vi "Test.vi"() -> ()   [LabVIEW 2020]
uses:
  g_industrial_cam/Device Enumeration.ctl
  g_industrial_cam/Camera/Camera.lvclass/Camera.ctl
  g_industrial_cam/Buffer/Buffer.lvclass/Buffer.ctl
  g_industrial_cam/Buffer/Create from Handle.vi
  g_industrial_cam/Camera/Check Not Disconnected.vi
  <vilib>/Utility/error.llb/Error Cluster From Error Code.vi
  <vilib>/picture/picture.llb/Draw 8-Bit Pixmap.vi
  g_industrial_cam/Buffer/Buffer.lvclass
  g_industrial_cam/Camera/Camera.lvclass
panel:
  out "Waveform Chart":i32(graph)
  out "Timeout":bool
  out "Devices":T1[](array[typedef])
  in  "Picture Zoom Factor":sgl
  out "2D Picture":picture
  out "Snap Shot Count":i32
  in  "stop":bool
  out "error out":errorcluster
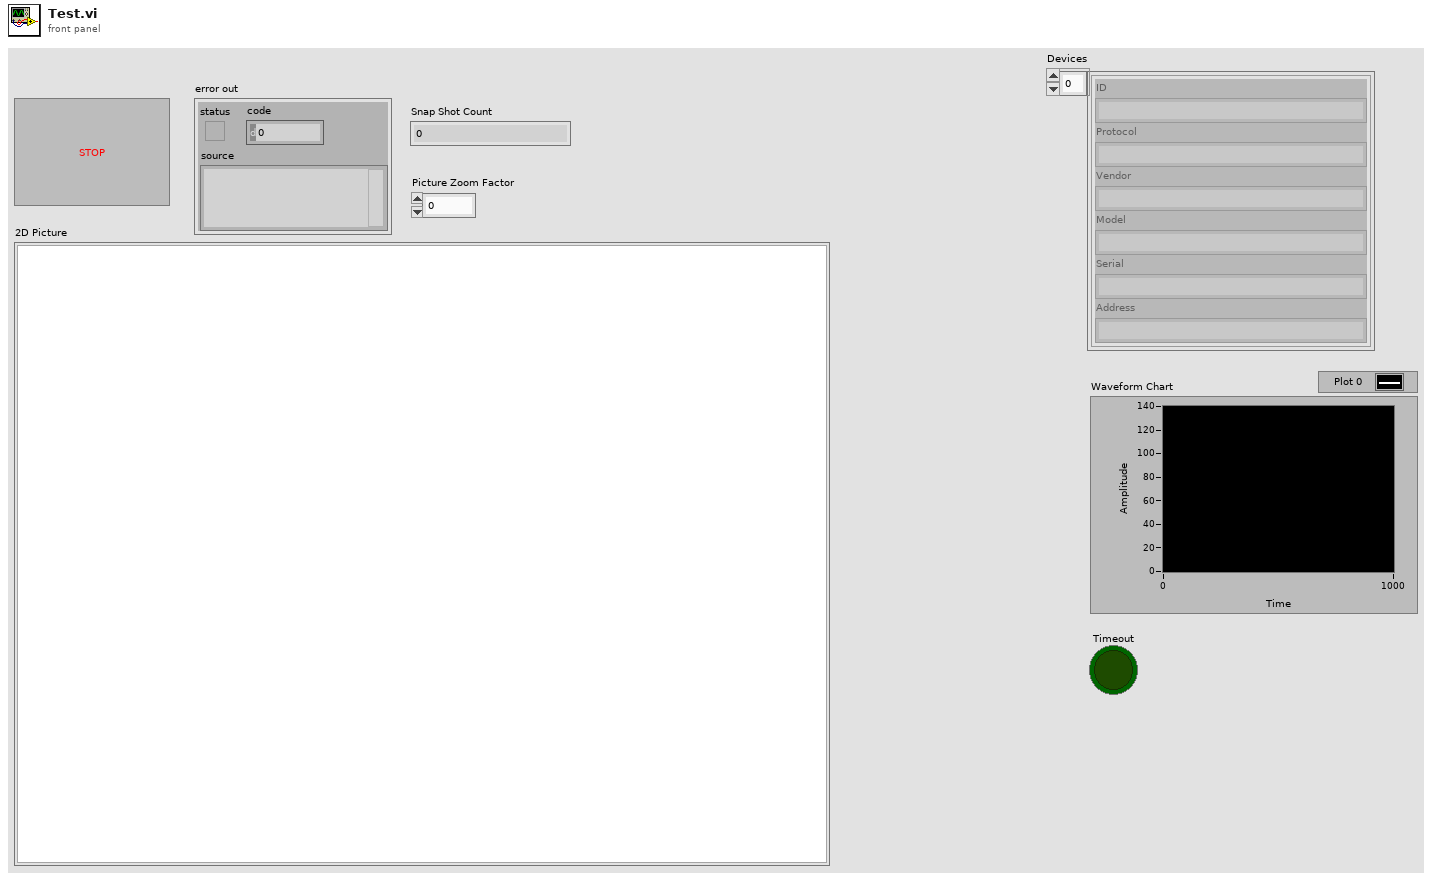
[diagram p1: front panel]
types:
  T1 = typedef "Device Enumeration.ctl" = cluster{"ID":string, "Protocol":string, "Vendor":string, "Model":string, "Serial":string, "Address":string}
  T2 = typedef "Buffer.lvclass/Image Size.ctl" = cluster{"Width":u16, "Height":u16}
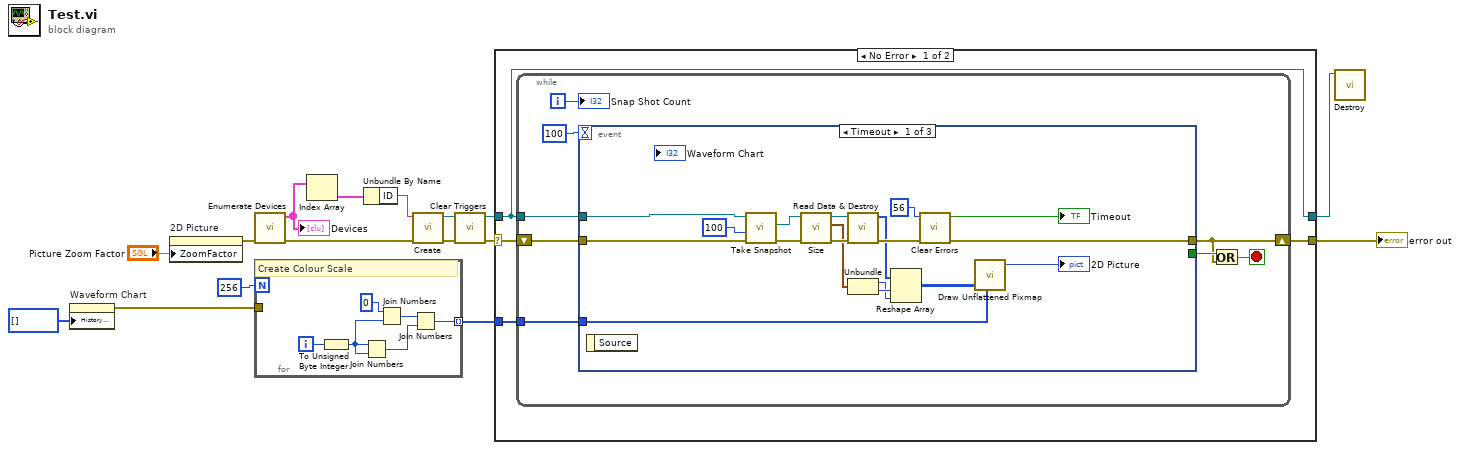
[diagram p0: block diagram]
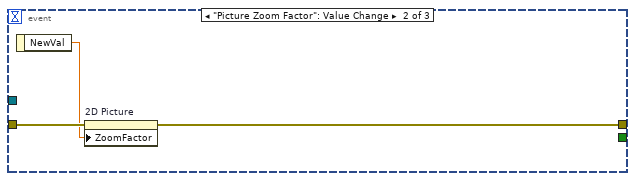
[diagram p2: hidden frame]
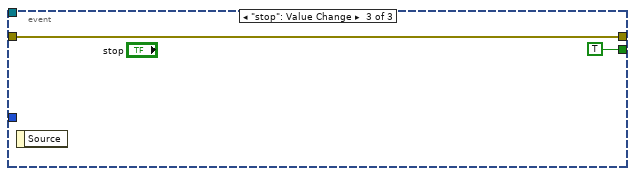
[diagram p3: hidden frame]
diagram:
  n1 = property on="Waveform Chart" class="WFChart (strict)"("History Data"=i32[] []) -> (error out=w5:errorcluster)  [unwired: 2 in, 1 out]
  n2 = property on="2D Picture" class="Pict"("ZoomFactor"="Picture Zoom Factor") -> (error out=w7:errorcluster)  [unwired: 2 in, 1 out]
  n3 = call "Enumerate Devices.vi"("error in (no error)"=w7) -> ("error out"=w14:errorcluster, "Devices"=w16:T1[])  [unwired: 9 in]
  "Devices" <- w16
  n4 = for {
    N: 256 -> [_]
    tunnel: [w17] -> w8 mode=indexing
    tunnel: w5 -> [_]
    i -> [w22]
    # "Create Colour Scale"
    n5 = To Unsigned Byte Integer(number=w22) -> (unsigned 8bit integer=w21:u8)
    n6 = Join Numbers(hi=w21, lo=w21) -> ((hi.lo)=w18:u16)
    n7 = Join Numbers(hi=u8 0, lo=w21) -> ((hi.lo)=w19:u16)
    n8 = Join Numbers(hi=w19, lo=w18) -> ((hi.lo)=w17:u32)
  }
  n9 = Index Array(array=w16) -> (element=w15:T1)  [unwired: 1 in]
  n10 = Unbundle By Name(w15) -> ("ID"=w13:string)
  n11 = call "Create.vi"("error in (no error)"=w14, "Identifier (ID, IP etc)"=w13) -> ("error out"=w12:errorcluster, "Camera"=w2:refnum<class "Camera.lvclass">)  [unwired: 8 in]
  n12 = call "Clear Triggers.vi"("error in (no error)"=w12, "Camera in"=w2) -> ("error out"=w3:errorcluster, "Camera"=w1:refnum<class "Camera.lvclass">)  [unwired: 8 in]
  n13 = case shown="No Error" w3 {
    selector: w3 -> [w26 w58]
    tunnel: w1 -> [w24 w59]
    tunnel: [w25 w58] -> w11
    tunnel: [w24 w59] -> w10
    tunnel: w8 -> [w23 _]
    frame No Error {
      n14 = while {
        shift-right: [w28] -> w25
        shift-left: w26 -> [w33]
        tunnel: w24 -> [w34]
        tunnel: w23 -> [w27]
        i -> [w30]
        stop <- w29 stop-if-true
        n15 = event shown="[0] Timeout" {
          selector: _ -> [_ _ _]
          dyn-events: _ -> [_ _ _]
          timeout: 100 -> [_ _ _]
          tunnel: w34 -> [w52 _ _]
          tunnel: w33 -> [w51 w55 w57]
          tunnel: [w50 w54 w57] -> w28
          tunnel: [_ _ TRUE] -> w32
          tunnel: w27 -> [w49 _ _]
          event Timeout {
            n16 = event-data() -> ()  [unwired: 1 in, 1 out]
            n17 = call "Take Snapshot.vi"("error in (no error)"=w51, "Timeout (ms)"=100, "Camera in"=w52) -> ("error out"=w45:errorcluster, "New Buffer"=w46:refnum<class "Buffer.lvclass">)  [unwired: 6 in, 1 out]
            n18 = call "Size.vi"("error in (no error)"=w45, "Buffer Data in"=w46) -> ("error out"=w44:errorcluster, "Image Size"=w42:T2, "Buffer Data"=w43:refnum<class "Buffer.lvclass">)  [unwired: 7 in]
            n19 = call "Read Data & Destroy.vi"("error in (no error)"=w44, "Buffer in"=w43) -> ("error out"=w39:errorcluster, "Data"=w38:u8[])  [unwired: 8 in]
            n20 = Unbundle(w42) -> ("Width"=w40:u16, "Height"=w41:u16)
            n21 = Reshape Array(w38, w41, w40) -> (w37:u8[][])
            n22 = call <vilib>:"Clear Errors.vi"("error in (no error)"=w39, "specific error code to clear (0: all)"=56) -> ("error out"=w50:errorcluster, "specific error cleared?"=→"Timeout":bool)  [unwired: 4 in]
            n23 = call-poly <vilib>:"Draw Unflattened Pixmap.vi"("data"=w37, "color table"=w49) -> ("new picture"=→"2D Picture":picture)  [unwired: 7 in]
          }
          event "Picture Zoom Factor": Value Change {
            n24 = event-data() -> ("NewVal"=w53:sgl)  [unwired: 1 in]
            n25 = property on="2D Picture" class="Pict"(error in=w55, "ZoomFactor"=w53) -> (error out=w54:errorcluster)  [unwired: 1 in, 1 out]
          }
          event "stop": Value Change {
            n26 = event-data() -> ()  [unwired: 1 in, 1 out]
          }
        }
        n27 = Or(x=w32, y=w28) -> (x .or. y?=w29:bool)
        "Snap Shot Count" <- w30
      }
    }
    frame Error {
    }
  }
  "error out" <- w11
  n28 = call "Destroy.vi"("Camera in"=w10) -> ()  [unwired: 10 in, 1 out]
